vi "Access Privilege_Remove Zero.vi"(7 "Input Array":u8[](array[numeric])) -> (8 "Output Array":u8[](array[numeric]))   [LabVIEW 2023, in "GUI.lvlib"]
doc: "Remove Zeros from Encrypted Data"
uses:
  GUI.lvlib
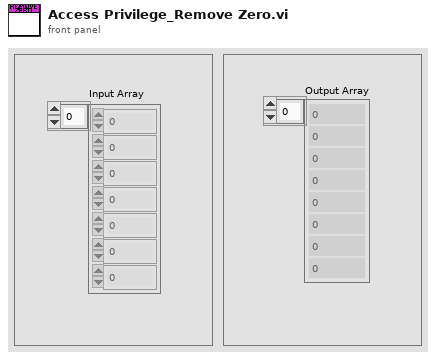
[diagram p1: front panel]
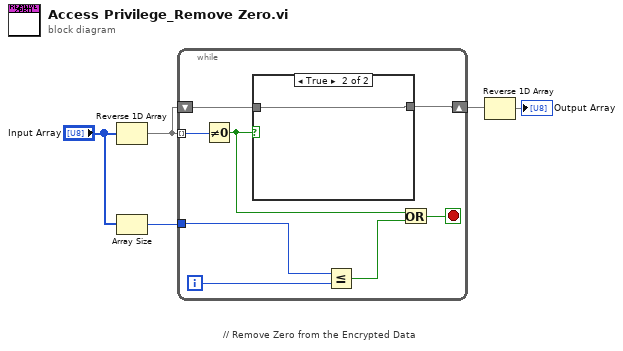
[diagram p0: block diagram]
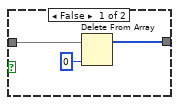
[diagram p2: hidden frame]
diagram:
  # "// Remove Zero from the Encrypted Data"
  n1 = Reverse 1D Array(array="Input Array") -> (reversed array=w5:u8[])
  n2 = Array Size(array="Input Array") -> (size(s)=w1:i32)
  n3 = while {
    tunnel: w5 -> [w13] mode=indexing
    shift-right: [w11] -> w4
    shift-left: w5 -> [w12]
    tunnel: w1 -> [w9]
    i -> [w8]
    stop <- w7 stop-if-true
    n4 = Not Equal To 0?(x=w13) -> (x != 0?=w10:bool)
    n5 = case shown="True" w10 {
      tunnel: w12 -> [w16 w17]
      tunnel: [w15 w17] -> w11
      frame False {
        n6 = Delete From Array(array=w16, index=0) -> (array with subset deleted=w15:u8[])  [unwired: 1 in, 1 out]
      }
      frame True {
      }
    }
    n7 = Less Or Equal?(x=w9, y=w8) -> (x <= y?=w6:bool)
    n8 = Or(x=w10, y=w6) -> (x .or. y?=w7:bool)
  }
  n9 = Reverse 1D Array(array=w4) -> (reversed array=→"Output Array":u8[])
